vi "FeuRouge.vi"() -> ()   [LabVIEW 2018]
uses:
  FeuRougeVar.vi
panel:
  in  "?":bool
  out "green":bool
  out "orange":bool
  out "red":bool
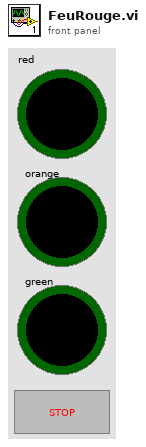
[diagram p1: front panel]
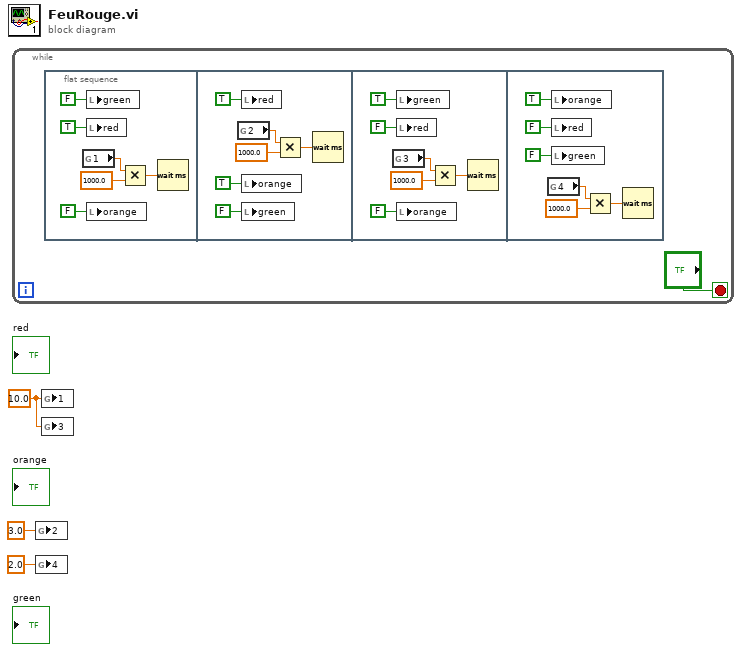
[diagram p0: block diagram]
diagram:
  w3 = 10.0 ("1")
  n1 = while {
    stop <- "?" stop-if-true
    n2 = flat-sequence {
      frame #0 {
        n3 = global read "FeuRougeVar.vi" "1"() -> (w10:dbl)
        n4 = local write "green"(FALSE) -> ()
        n5 = local write "red"(TRUE) -> ()
        n6 = local write "orange"(FALSE) -> ()
        n7 = Multiply(x=w10, y=1000.0) -> (x*y=w8:dbl)
        n8 = Wait (ms)(milliseconds to wait=w8) -> ()  [unwired: 1 out]
      }
      frame #1 {
        n9 = global read "FeuRougeVar.vi" "2"() -> (w15:dbl)
        n10 = local write "red"(TRUE) -> ()
        n11 = local write "orange"(TRUE) -> ()
        n12 = local write "green"(FALSE) -> ()
        n13 = Multiply(x=w15, y=1000.0) -> (x*y=w16:dbl)
        n14 = Wait (ms)(milliseconds to wait=w16) -> ()  [unwired: 1 out]
      }
      frame #2 {
        n15 = global read "FeuRougeVar.vi" "3"() -> (w21:dbl)
        n16 = local write "green"(TRUE) -> ()
        n17 = local write "red"(FALSE) -> ()
        n18 = local write "orange"(FALSE) -> ()
        n19 = Multiply(x=w21, y=1000.0) -> (x*y=w20:dbl)
        n20 = Wait (ms)(milliseconds to wait=w20) -> ()  [unwired: 1 out]
      }
      frame #3 {
        n21 = global read "FeuRougeVar.vi" "4"() -> (w27:dbl)
        n22 = local write "orange"(TRUE) -> ()
        n23 = local write "red"(FALSE) -> ()
        n24 = local write "green"(FALSE) -> ()
        n25 = Multiply(x=w27, y=1000.0) -> (x*y=w28:dbl)
        n26 = Wait (ms)(milliseconds to wait=w28) -> ()  [unwired: 1 out]
      }
    }
  }
  n27 = global write "FeuRougeVar.vi" "2"(3.0 ("2")) -> ()
  n28 = global write "FeuRougeVar.vi" "4"(2.0 ("4")) -> ()
  n29 = global write "FeuRougeVar.vi" "1"(w3) -> ()
  n30 = global write "FeuRougeVar.vi" "3"(w3) -> ()
